vi "Get Wire Selected Parts Bounds.vi"(8 "error in":errorcluster, 11 "Wire in":refnum<vi>) -> (0 "error out":errorcluster, 2 "Selected Parts Bounds":T1, 3 "Wire out":refnum<vi>)   [LabVIEW 2020, in "Enclose in Structure.lvlib"]
uses:
  Enclose in Structure.lvlib
  <vilib>/Utility/miscctls.llb/LVRectTypeDef.ctl
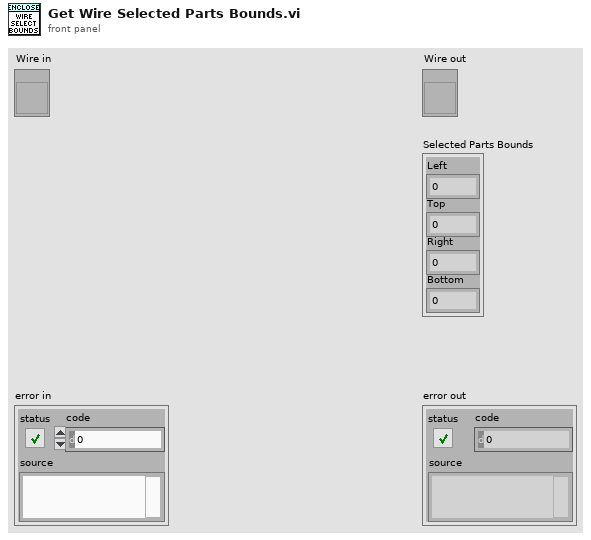
[diagram p1: front panel]
types:
  T1 = typedef "LVRectTypeDef.ctl" = cluster{"Left":i16, "Top":i16, "Right":i16, "Bottom":i16}
  T2 = cluster{"Position":cluster{"h":i16, "v":i16}, "Flags":i32, "Type":enum32{"LooseEnd", "Endpoint", "Bend", "Junction"}, "Up Joint Index":i16, "Down Joint Index":i16, "Left Joint Index":i16, "Right Joint Index":i16}[]
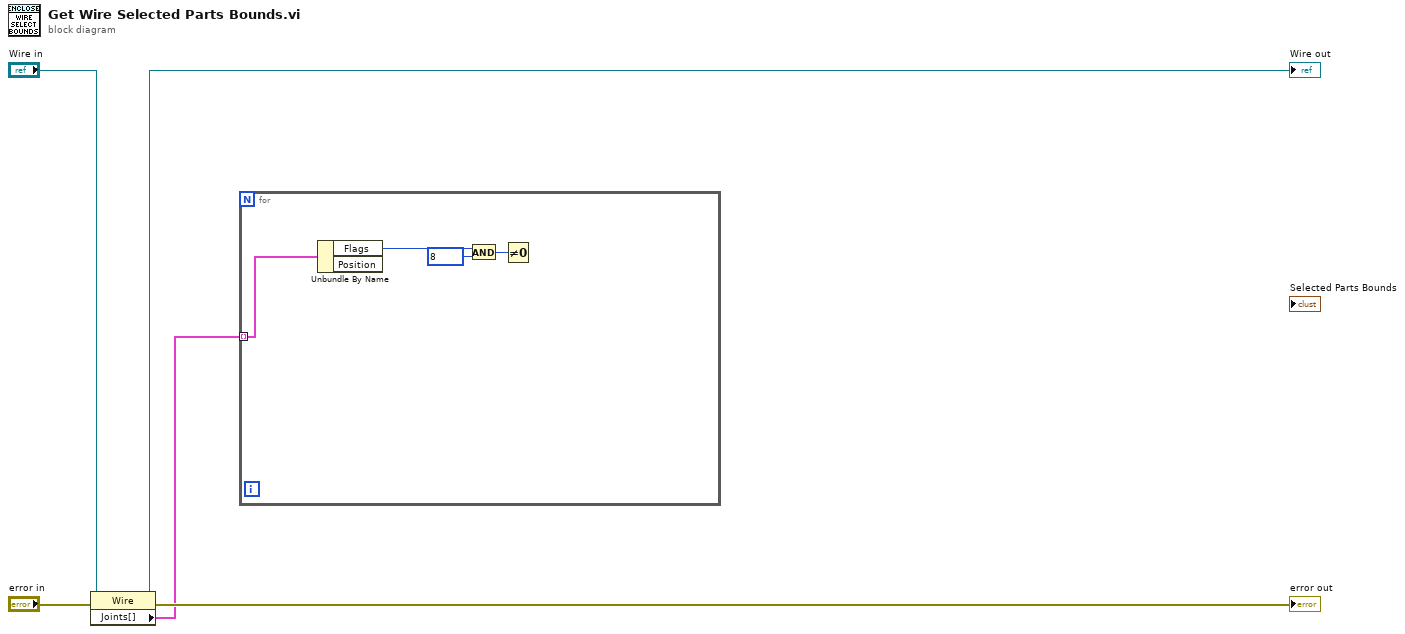
[diagram p0: block diagram]
diagram:
  n1 = property class="Wire"(reference="Wire in", error in="error in") -> (reference out=→"Wire out":refnum<vi>, error out=→"error out":errorcluster, "Joints[]"=w3:T2)
  n2 = for {
    tunnel: w3 -> [w9] mode=indexing
    n3 = Unbundle By Name(w9) -> ("Flags"=w8:i32)  [unwired: 1 out]
    n4 = And(x=w8, y=8) -> (x .and. y?=w6:i32)
    n5 = Not Equal To 0?(x=w6) -> ()  [unwired: 1 out]
  }
